vi "TSFL1dll.vi"(8 "error in (no error)":errorcluster, 11 "Inputs":T2) -> (0 "error out":errorcluster, 3 "Outputs":T1)   [LabVIEW 2016]
uses:
  REFPROP.DLL
panel:
  # "REFPROP-TSFL1dll.vi"
  # "void  TSFL1dll(double *t, double *s, double *z, double *dmin, double dmax, double d, int32_t *ierr, CStr herr, int32_t herr_length);"
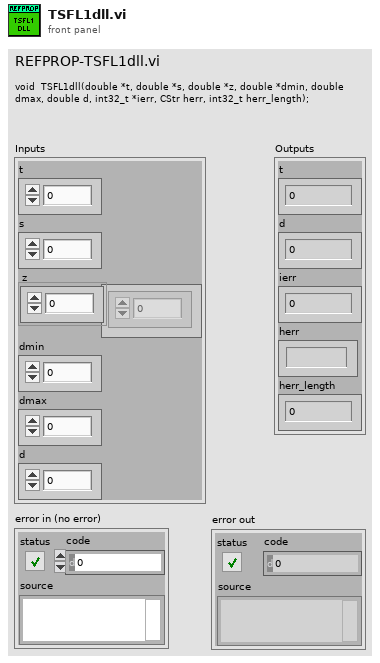
[diagram p1: front panel]
types:
  T1 = cluster{"t":dbl, "d":dbl, "ierr":i32, "herr":string, "herr_length":i32}
  T2 = cluster{"t":dbl, "s":dbl, "z":dbl[], "dmin":dbl, "dmax":dbl, "d":dbl}
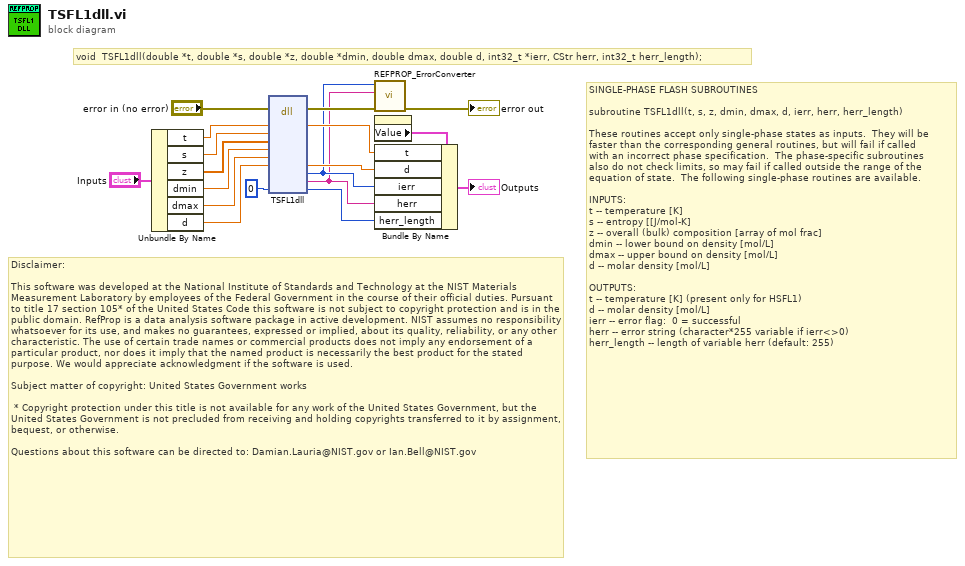
[diagram p0: block diagram]
diagram:
  # "Disclaimer:\n\nThis software was developed at the National Institute of Standards and Technology at the NIST Materials Measurement Laboratory by employees of the Federal Government in the course of their official duties. Pursuant to title 17 section 105* of the United States Code this software is not subject to copyright protection and is in the public domain. RefProp is a data analysis software package in active development. NIST assumes no responsibility whatsoever for its use, and makes no guarantees, expressed or implied, about its quality, reliability, or any other characteristic. The use of certain trade names or commercial products does not imply any endorsement of a particular product, nor does it imply that the named product is necessarily the best product for the stated purpose. We would appreciate acknowledgment if the software is used.\n \nSubject matter of copyright: United States Government works\n  \n * Copyright protection under this title is not available for any work of the United States Government, but the United States Government is not precluded from receiving and holding copyrights transferred to it by assignment, bequest, or otherwise.\n\nQuestions about this software can be directed to: Damian.Lauria@NIST.gov or Ian.Bell@NIST.gov"
  # "void  TSFL1dll(double *t, double *s, double *z, double *dmin, double dmax, double d, int32_t *ierr, CStr herr, int32_t herr_length);"
  # "SINGLE-PHASE FLASH SUBROUTINES\n\nsubroutine TSFL1dll(t, s, z, dmin, dmax, d, ierr, herr, herr_length) \n\nThese routines accept only single-phase states as inputs.  They will be\nfaster than the corresponding general routines, but will fail if called\nwith an incorrect phase specification.  The phase-specific subroutines\nalso do not check limits, so may fail if called outside the range of the\nequation of state.  The following single-phase routines are available.\n\nINPUTS: \nt -- temperature [K]\ns -- entropy [[J/mol-K]\nz -- overall (bulk) composition [array of mol frac]\ndmin -- lower bound on density [mol/L]\ndmax -- upper bound on density [mol/L]\nd -- molar density [mol/L]\n\nOUTPUTS:\nt -- temperature [K] (present only for HSFL1)\nd -- molar density [mol/L]\nierr -- error flag:  0 = successful\nherr -- error string (character*255 variable if ierr<>0)\nherr_length -- length of variable herr (default: 255)"
  n1 = Unbundle By Name("Inputs") -> ("t"=w11:dbl, "s"=w10:dbl, "z"=w9:dbl[], "dmin"=w8:dbl, "dmax"=w7:dbl, "d"=w6:dbl)
  n2 = dll-call lib="S:/009 - Testing/02 - Performance Testing/REFPROP/REFPROP.*" fn="TSFL1dll"(error in="error in (no error)", "t"=w11, "s"=w10, "z"=w9, "dmin"=w8, "dmax"=w7, "d"=w6, "herr_length"=0) -> (error out=w13:errorcluster, "t"=w5:dbl, "d"=w4:dbl, "ierr"=w3:i32, "herr"=w2:string, "herr_length"=w1:i32)  [unwired: 9 in, 1 out]
  n3 = call "REFPROP_ErrorConverter.vi"("error in (no error)"=w13, "Error Message"=w2, "Error Code"=w3) -> ("error out"=→"error out":errorcluster)  [unwired: 8 in]
  n4 = property on="Outputs" class="Clust (strict)"() -> ("Value"=w16:T1)  [unwired: 2 in, 2 out]
  n5 = Bundle By Name(cluster=w16, "t"=w5, "d"=w4, "ierr"=w3, "herr"=w2, "herr_length"=w1) -> (→"Outputs":T1)
